vi "Next Available Datum Index.vi"(1 "bytestream":refnum<class "Bytestream.lvclass">) -> (0 "index":i32)   [LabVIEW 2020, in "NI_Bytestream.lvlib" / "Bytestream.lvclass"]
uses:
  <vilib>/Array/Bytestream/Bytestream.lvclass
  <vilib>/Array/Bytestream/Bytestream.lvclass/Bytestream.ctl
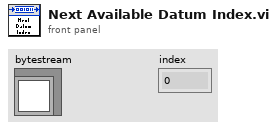
[diagram p1: front panel]
types:
  T1 = typedef "NI_Bytestream.lvlib/Bytestream.lvclass/Datum.ctl" = cluster{"array":u8[], "index":i32}
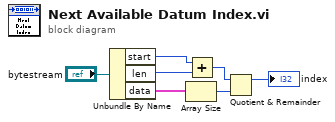
[diagram p0: block diagram]
diagram:
  n1 = Unbundle By Name("bytestream") -> ("start"=w6:i32, "len"=w5:i32, "data"=w4:T1[])
  n2 = Array Size(array=w4) -> (size(s)=w2:i32)
  n3 = Add(x=w6, y=w5) -> (x+y=w3:i32)
  n4 = Quotient & Remainder(x=w3, y=w2) -> (x-y*floor(x/y)=→"index":i32)  [unwired: 1 out]
